vi "Video record flag cleanup.vi"   [LabVIEW 2013]
uses:
  typedefs/Functions enum.ctl
types:
  T1 = typedef "Functions enum.ctl" = enum16{"Create", "Start", "Write", "Stop", "Clear"}
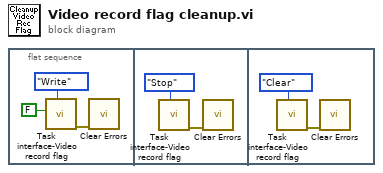
[diagram p0: block diagram]
diagram:
  n1 = flat-sequence {
    frame #0 {
      n2 = call "Task interface-Video record flag.vi"("Function"=Functions_enum."Write", "DO value"=FALSE) -> ("error out"=w1:errorcluster)  [unwired: 9 in]
      n3 = call <vilib>:"Clear Errors.vi"("error in (no error)"=w1) -> ()  [unwired: 6 in, 1 out]
    }
    frame #1 {
      n4 = call "Task interface-Video record flag.vi"("Function"=Functions_enum."Stop") -> ("error out"=w4:errorcluster)  [unwired: 10 in]
      n5 = call <vilib>:"Clear Errors.vi"("error in (no error)"=w4) -> ()  [unwired: 6 in, 1 out]
    }
    frame #2 {
      n6 = call "Task interface-Video record flag.vi"("Function"=Functions_enum."Clear") -> ("error out"=w6:errorcluster)  [unwired: 10 in]
      n7 = call <vilib>:"Clear Errors.vi"("error in (no error)"=w6) -> ()  [unwired: 6 in, 1 out]
    }
  }
